vi "RunDuringExperiment_5_May_2014.vi"() -> ()   [LabVIEW 2012]
uses:
  GlobalVars.vi
panel:
  out "Elements in Data Queue":i32
  in  "Average N Reference Frames":dbl=1.0 min=1.0
  in  "Position Shift Limit (Microns)":dbl=3.0 min=0.0
  out "Out of Limits":bool
  out "Z1":waveform(dbl)(graph)
  out "Y1":waveform(dbl)(graph)
  out "X1":waveform(dbl)(graph)
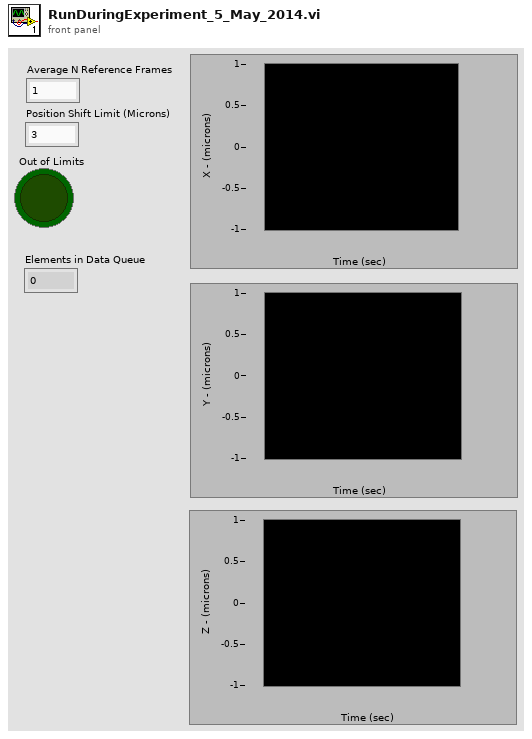
[diagram p1: front panel]
types:
  T1 = cluster{"gridsize":u16, "data":i32[][], "coordinates":i32[][], "settings":i32[], "settings_um":i32[], "needsreference":bool}
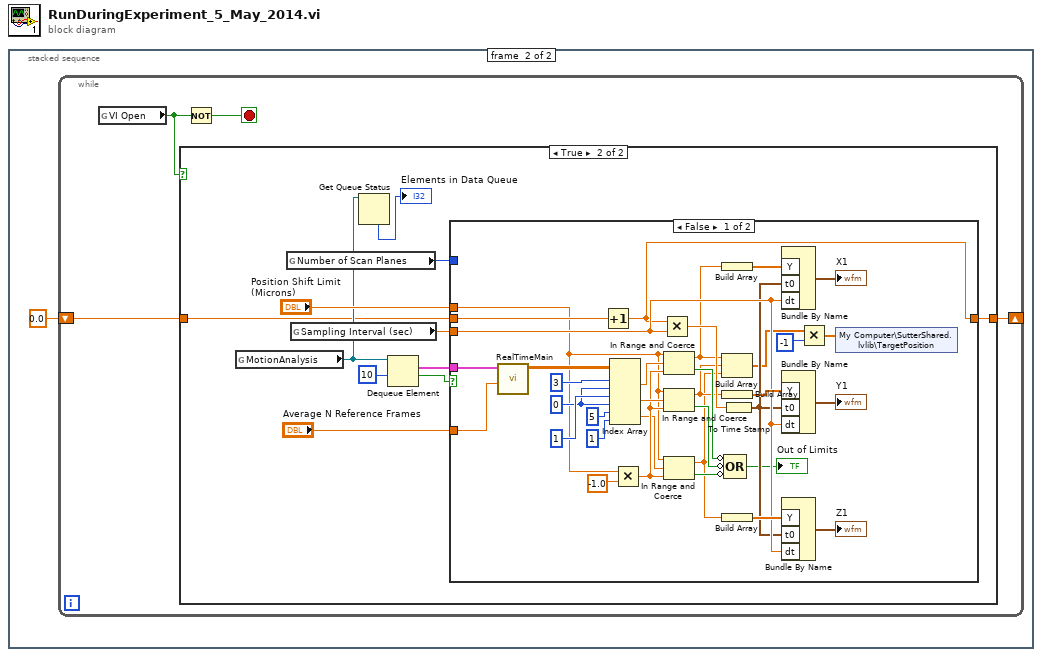
[diagram p0: block diagram]
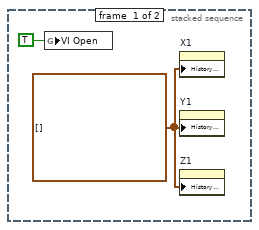
[diagram p2: hidden frame]
diagram:
  n1 = stacked-sequence {
    frame #0 {
      w1 = waveform(dbl)[] [] ("History Data")
      n2 = global write "GlobalVars.vi" "VI Open"(TRUE ("VI Open")) -> ()
      n3 = property on="X1" class="WFChart (strict)"("History Data"=w1) -> ()  [unwired: 2 in, 2 out]
      n4 = property on="Y1" class="WFChart (strict)"("History Data"=w1) -> ()  [unwired: 2 in, 2 out]
      n5 = property on="Z1" class="WFChart (strict)"("History Data"=w1) -> ()  [unwired: 2 in, 2 out]
    }
    frame #1 {
      n6 = while {
        shift-right: [w4] -> _
        shift-left: 0.0 -> [w5]
        stop <- w7 stop-if-true
        n7 = global read "GlobalVars.vi" "VI Open"() -> (w6:bool)
        n8 = case shown="True" w6 {
          tunnel: w5 -> [w8 w11]
          tunnel: [w8 w10] -> w4
          frame False {
          }
          frame True {
            n9 = global read "GlobalVars.vi" "MotionAnalysis"() -> (w13:refnum<queue>)
            n10 = global read "GlobalVars.vi" "Number of Scan Planes"() -> (w16:i32)
            n11 = global read "GlobalVars.vi" "Sampling Interval (sec)"() -> (w9:dbl)
            n12 = Get Queue Status(queue=w13) -> (# elements in queue=→"Elements in Data Queue":i32)  [unwired: 2 in, 7 out]
            n13 = Dequeue Element(queue=w13, timeout in ms (-1)=10) -> (element=w17:T1, timed out?=w15:bool)  [unwired: 1 in, 2 out]
            n14 = case shown="False" w15 {
              tunnel: "Position Shift Limit (Microns)" -> [w31 _]
              tunnel: "Average N Reference Frames" -> [w54 _]
              tunnel: w17 -> [w53 _]
              tunnel: w16 -> [_ _]
              tunnel: w9 -> [w38 _]
              tunnel: w11 -> [w40 w55]
              tunnel: [w37 w55] -> w10
              frame False {
                w48 = 0 ("disabled index (col)")
                n15 = call "RealTimeMain.vi"("For Reference (frames)"=w54, "Motion Data"=w53) -> ("Array"=w52:dbl[][])  [unwired: 9 in]
                n16 = Increment(x=w40) -> (x+1=w37:dbl)
                n17 = Index Array(array=w52, index (row) #1=3 ("index (row)"), index (col) #1=w48, index (row) #2=1 ("index (row)"), index (col) #2=w48, index (row) #3=5 ("index (row)"), index (col) #3=1 ("disabled index (col)")) -> (element #1=w34:dbl, element #2=w33:dbl, element #3=w30:dbl)
                n18 = Multiply(x=w31, y=-1.0) -> (x*y=w32:dbl)
                n19 = Multiply(x=w37, y=w38) -> (x*y=w39:dbl)
                n20 = In Range and Coerce(upper limit=w31, x=w34, lower limit=w32) -> (coerced(x)=w25:dbl, In Range?=w29:bool)
                n21 = In Range and Coerce(upper limit=w31, x=w33, lower limit=w32) -> (coerced(x)=w24:dbl, In Range?=w28:bool)
                n22 = In Range and Coerce(upper limit=w31, x=w30, lower limit=w32) -> (coerced(x)=w23:dbl, In Range?=w27:bool)
                n23 = Build Array(w25) -> (w45:dbl[])
                n24 = Build Array(w25, w24, w23) -> (w22:dbl[])
                n25 = Build Array(w24) -> (w41:dbl[])
                n26 = Build Array(w23) -> (w42:dbl[])
                n27 = To Time Stamp(1:w39) -> (0:w36:timestamp)
                n28 = Compound Arithmetic op=OR(invert w29, invert w28, invert w27) -> (→"Out of Limits":bool)
                n29 = Bundle By Name("Y"=w45, "t0"=w36, "dt"=w38) -> (→"X1":waveform(dbl))  [unwired: 1 in]
                n30 = Bundle By Name("Y"=w41, "t0"=w36, "dt"=w38) -> (→"Y1":waveform(dbl))  [unwired: 1 in]
                n31 = Bundle By Name("Y"=w42, "t0"=w36, "dt"=w38) -> (→"Z1":waveform(dbl))  [unwired: 1 in]
                n32 = Multiply(x=w22, y=-1) -> (x*y=w20:dbl[])
                n33 = shared-variable "My Computer\\SutterShared.lvlib\\TargetPosition"(w20) -> ()  [unwired: 1 in, 1 out]
              }
              frame True {
              }
            }
          }
        }
        n34 = Not(x=w6) -> (.not. x?=w7:bool)
      }
    }
  }
